vi "Create From Variant.vi"(8 "error in (no error)":errorcluster, 10 "Variant":variant, 11 "JSON Boolean in":refnum<class "JSON Boolean.lvclass">) -> (0 "error out":errorcluster, 3 "JSON Boolean out":refnum<class "JSON Boolean.lvclass">)   [LabVIEW 2015, in "LVJSON.lvlib" / "JSON Boolean.lvclass"]
uses:
  JSON Boolean.lvclass
  JSON Boolean.lvclass/JSON Boolean.ctl
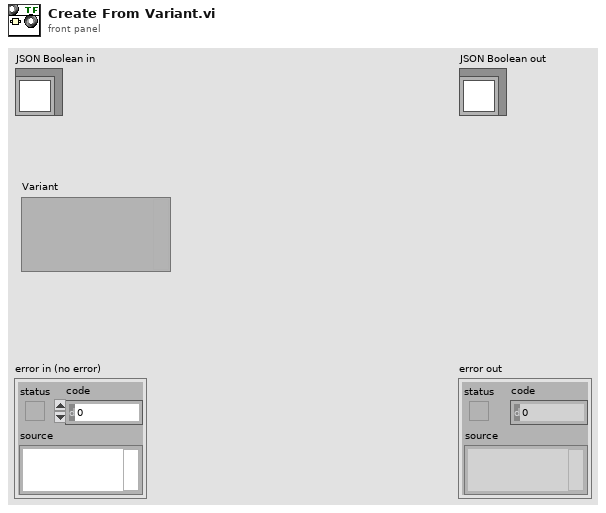
[diagram p1: front panel]
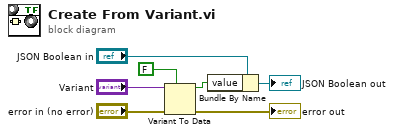
[diagram p0: block diagram]
diagram:
  n1 = Variant To Data(error in="error in (no error)", type=FALSE, Variant="Variant") -> (data=w4:bool, error out=→"error out":errorcluster)
  n2 = Bundle By Name(cluster="JSON Boolean in", "value"=w4) -> (→"JSON Boolean out":refnum<class "JSON Boolean.lvclass">)
